vi "Load Colors.vi"(1 "Viewer Path":path) -> (0 "Color Names & Values":T1)   [LabVIEW 2015, in "GraphViz Mapping Visualizer.lvlib"]
doc: "Loads a X11 html table from File (Else uses default colours).\nNote X11 table had white font tags and &nbsp; removed. \nReturns default color names and their RGB color box values."
uses:
  GraphViz Mapping Visualizer.lvlib
panel:
  out "Supported Colors":string[](array[string])
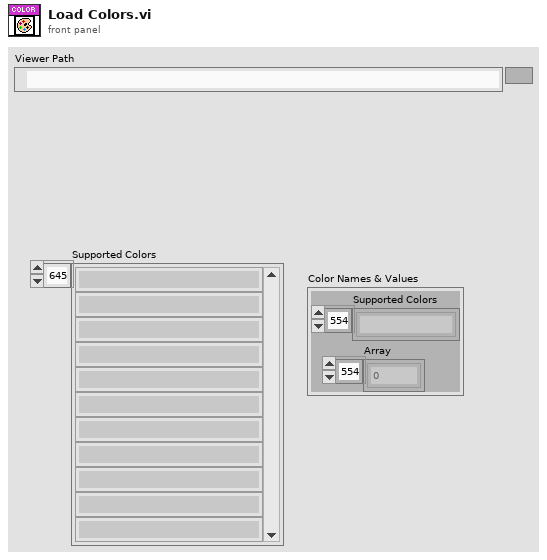
[diagram p1: front panel]
types:
  T1 = cluster{"Supported Colors":string[], "Array":u32[]}
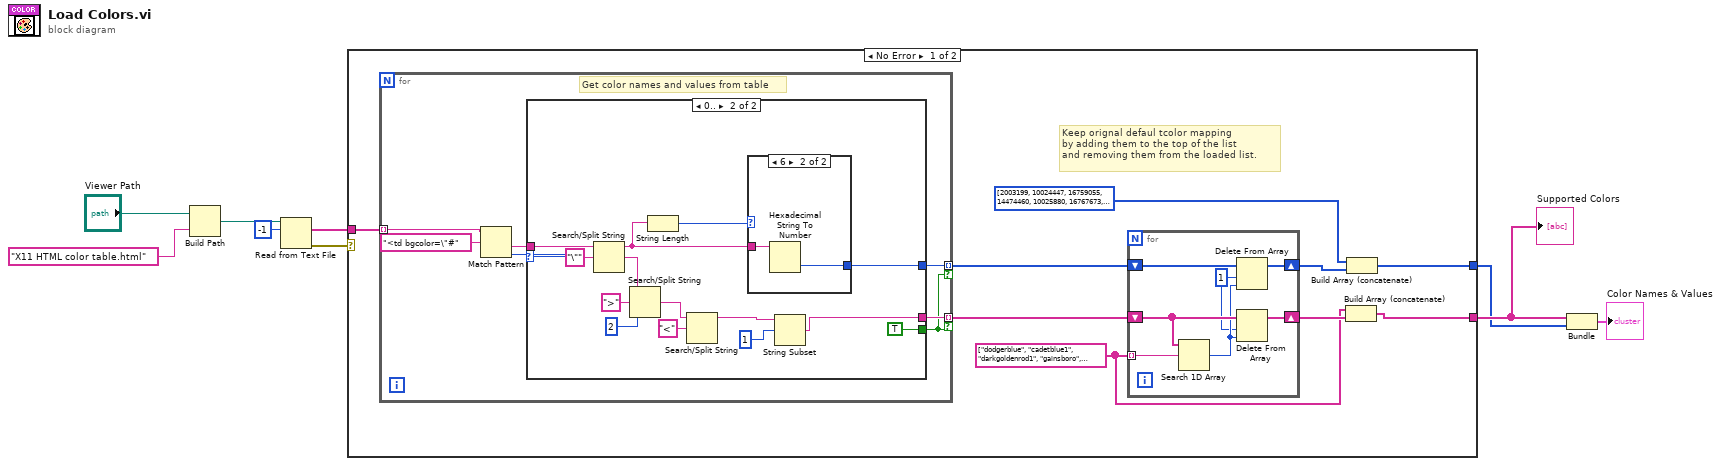
[diagram p0: block diagram]
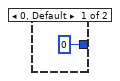
[diagram p3: hidden frame]
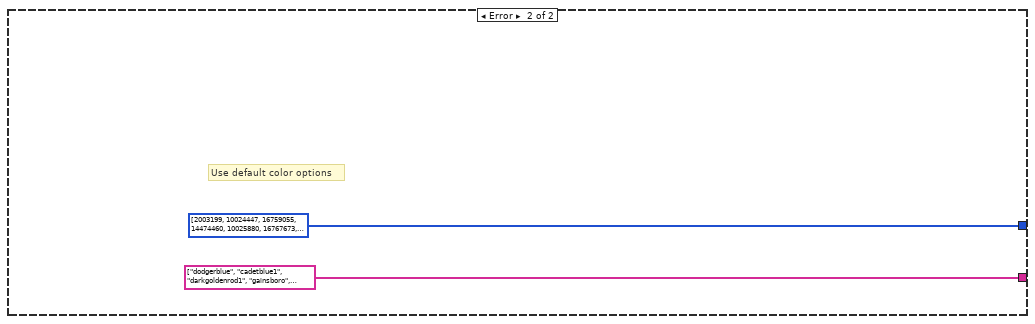
[diagram p4: hidden frame]
diagram:
  n1 = Build Path(base path="Viewer Path", name or relative path="X11 HTML color table.html") -> (appended path=w7:path)
  n2 = Read from Text File(file (use dialog)=w7, count=-1) -> (text=w4:string[], error out=w5:errorcluster)  [unwired: 2 in, 2 out]
  n3 = case shown="No Error" w5 {
    tunnel: w4 -> [w18 _]
    tunnel: [w11 string[] ["dodgerblue", "cadetblue1", "darkgoldenrod1", "gainsboro", "palegreen", "peachpuff", "violet", "skyblue", "yellow", "seagreen1", "tomato", "thistle", "slateblue1", "orange", "palevioletred1"] ("Supported Colors")] -> w3
    tunnel: [w10 u32[] [2003199, 10024447, 16759055, 14474460, 10025880, 16767673, 15631086, 8900331, 16776960, 5570463, 16737095, 14204888, 8613887, 16753920, 16745131] ("Array")] -> w2
    frame No Error {
      w12 = string[] ["dodgerblue", "cadetblue1", "darkgoldenrod1", "gainsboro", "palegreen", "peachpuff", "violet", "skyblue", "yellow", "seagreen1", "tomato", "thistle", "slateblue1", "orange", "palevioletred1"] ("Supported Colors")
      # "Keep orignal defaul tcolor mapping\nby adding them to the top of the list\nand removing them from the loaded list."
      n4 = for {
        tunnel: w18 -> [w32] mode=indexing
        tunnel: [w28] -> w16 mode=indexing if=w26
        tunnel: [w27] -> w17 mode=indexing if=w26
        # "Get color names and values from table"
        n5 = Match Pattern(string=w32, regular expression="<td bgcolor=\"#") -> (after substring=w29:string, offset past match=w30:i32)  [unwired: 1 in, 2 out]
        n6 = case shown="0.." w30 {
          tunnel: w29 -> [_ w46]
          tunnel: [_ w33] -> w28
          tunnel: [_ TRUE] -> w26
          tunnel: [_ w37] -> w27
          frame Default {
          }
          frame 0.. {
            n7 = Search/Split String(string=w46, search string/char (-)="\"") -> (substring before match=w43:string, match + rest of string=w36:string)  [unwired: 1 in, 1 out]
            n8 = Search/Split String(string=w36, search string/char (-)=">", offset (0)=2) -> (match + rest of string=w40:string)  [unwired: 2 out]
            n9 = String Length(string=w43) -> (length=w44:i32)
            n10 = Search/Split String(string=w40, search string/char (-)="<") -> (substring before match=w34:string)  [unwired: 1 in, 2 out]
            n11 = case shown="6" w44 {
              tunnel: w43 -> [_ w49]
              tunnel: [u32 0 w48] -> w37
              frame 0, Default {
              }
              frame 6 {
                n12 = Hexadecimal String To Number(string=w49) -> (number=w48:u32)  [unwired: 2 in, 1 out]
              }
            }
            n13 = String Subset(string=w34, offset (0)=1) -> (substring=w33:string)  [unwired: 1 in]
          }
        }
      }
      n14 = for {
        tunnel: w12 -> [w25] mode=indexing
        shift-right: [w20] -> w15
        shift-left: w17 -> [w23]
        shift-right: [w19] -> w13
        shift-left: w16 -> [w24]
        w21 = 1 ("length")
        n15 = Search 1D Array(1D array=w24, element=w25) -> (index of element=w22:i32)  [unwired: 1 in]
        n16 = Delete From Array(array=w23, length=w21, index=w22) -> (array with subset deleted=w20:u32[])  [unwired: 1 out]
        n17 = Delete From Array(array=w24, length=w21, index=w22) -> (array with subset deleted=w19:string[])  [unwired: 1 out]
      }
      n18 = Build Array (concatenate)(w12, w13) -> (w11:string[])
      n19 = Build Array (concatenate)(u32[] [2003199, 10024447, 16759055, 14474460, 10025880, 16767673, 15631086, 8900331, 16776960, 5570463, 16737095, 14204888, 8613887, 16753920, 16745131] ("Array"), w15) -> (w10:u32[])
    }
    frame Error {
      # "Use default color options"
    }
  }
  "Supported Colors" <- w3
  n20 = Bundle("Supported Colors"=w3, "Array"=w2) -> (→"Color Names & Values":T1)  [unwired: 1 in]
